vi "Limelight LED OFF.vi"(8 "error in (no error)":errorcluster, 11 "LED OFF (T)":bool) -> ()   [LabVIEW 2020]
uses:
  <vilib>/Rock Robotics/Network Tables/NT Write Number.vi
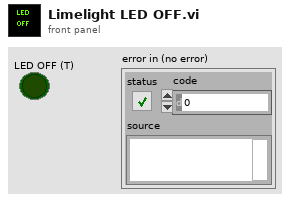
[diagram p1: front panel]
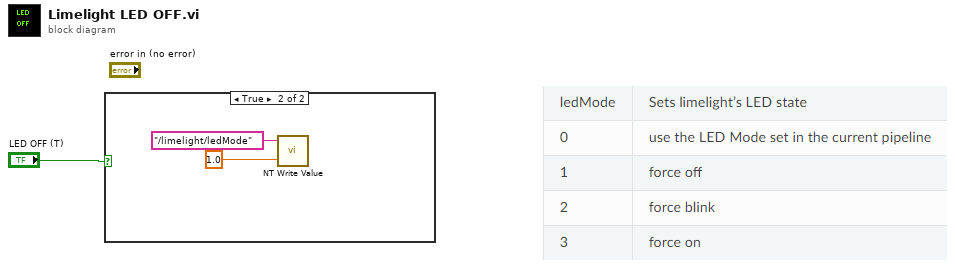
[diagram p0: block diagram]
diagram:
  n1 = case shown="True" "LED OFF (T)" {
    frame False {
    }
    frame True {
      n2 = call-poly <vilib>:"NT Write Value.vi"("Numeric"=1.0, "Name"="/limelight/ledMode") -> ()  [unwired: 9 in, 1 out]
    }
  }
